vi "EX382280_Interface.vi"(7 "mode":T1, 8 "error in (no error)":errorcluster caption="에러 입력(에러 없음)", 9 "Current(A)":dbl, 10 "Voltage(V)":dbl, 11 "VISA resource name":refnum<visa-resource-name> caption="Port") -> (0 "error out":errorcluster, 3 "Read":string)   [LabVIEW 2015]
uses:
  382280_mode.ctl
  <vilib>/Instr/_visa.llb/VISA Configure Serial Port (Serial Instr).vi
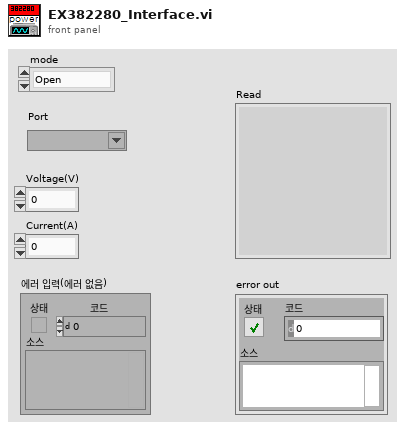
[diagram p1: front panel]
types:
  T1 = typedef "382280_mode.ctl" = enum16{"Open", "Close", "STBY", "OPER", "V SET", "A SET", "STATUS", "V Read", "A Read"}
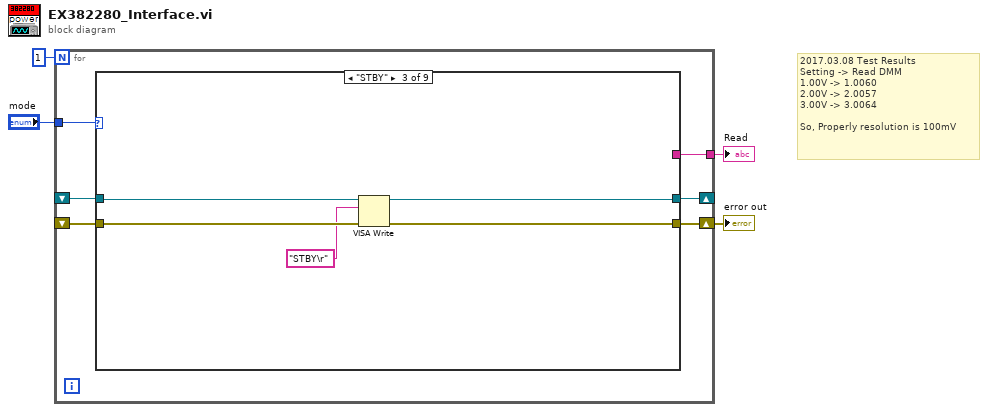
[diagram p0: block diagram]
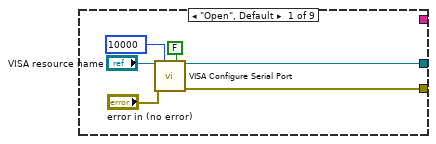
[diagram p2: hidden frame]
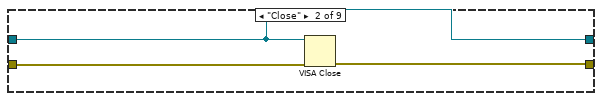
[diagram p3: hidden frame]
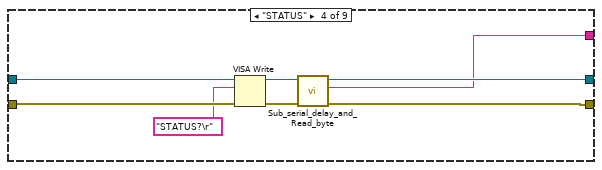
[diagram p4: hidden frame]
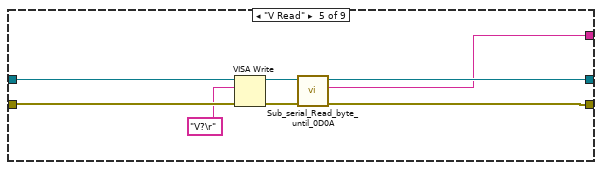
[diagram p5: hidden frame]
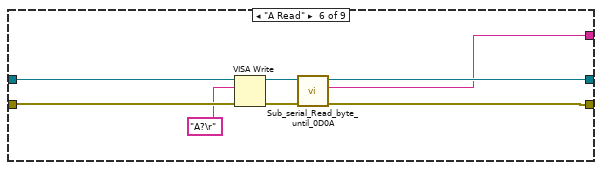
[diagram p6: hidden frame]
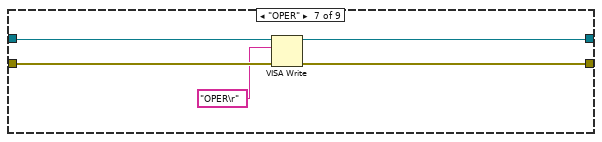
[diagram p7: hidden frame]
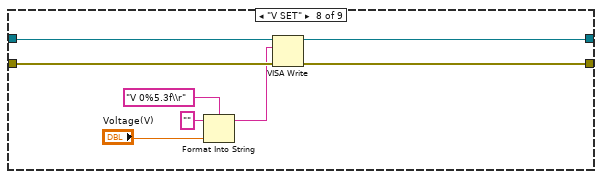
[diagram p8: hidden frame]
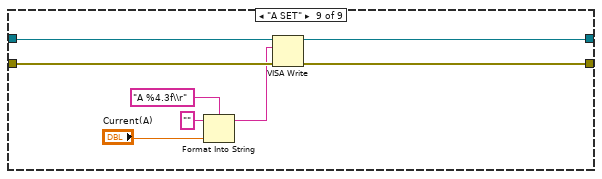
[diagram p9: hidden frame]
diagram:
  # "2017.03.08 Test Results\nSetting -> Read DMM\n1.00V -> 1.0060\n2.00V -> 2.0057 \n3.00V -> 3.0064\n\nSo, Properly resolution is 100mV"
  n1 = for {
    N: 1 -> [_]
    tunnel: "mode" -> [w10]
    shift-right: [w9] -> _
    shift-left: _ -> [w7]
    shift-right: [w8] -> w2
    shift-left: _ -> [w6]
    tunnel: [w5] -> w1
    n2 = case shown="\"STBY\"" w10 {
      tunnel: [w12 w18 w20 w32 w40 w48 w49 w56 w64] -> w9
      tunnel: [w11 w17 w22 w31 w39 w47 w51 w58 w66] -> w8
      tunnel: w7 -> [_ w18 w21 w29 w37 w45 w50 w57 w65]
      tunnel: w6 -> [_ w19 w24 w30 w38 w46 w53 w61 w69]
      tunnel: [_ _ _ w26 w34 w42 _ _ _] -> w5
      frame "Open", Default {
        n3 = call-poly "VISA Configure Serial Port"("VISA resource name"="VISA resource name", "timeout (10sec)"=u32 10000, "Enable Termination\nChar (T)"=FALSE ("Enable Termination\nChar (T)"), "error in (no error)"="error in (no error)") -> ("VISA resource name out"=w12:refnum<visa-resource-name>, "error out"=w11:errorcluster)  [unwired: 10 in]
      }
      frame "Close" {
        n4 = VISA Close(VISA resource name=w18, error in (no error)=w19) -> (error out=w17:errorcluster)
      }
      frame "STBY" {
        n5 = VISA Write(VISA resource name=w21, write buffer="STBY\r" ("버퍼 쓰기"), error in (no error)=w24) -> (VISA resource name out=w20:refnum<visa-resource-name>, error out=w22:errorcluster)  [unwired: 1 out]
      }
      frame "STATUS" {
        n6 = VISA Write(VISA resource name=w29, write buffer="STATUS?\r" ("버퍼 쓰기"), error in (no error)=w30) -> (VISA resource name out=w27:refnum<visa-resource-name>, error out=w28:errorcluster)  [unwired: 1 out]
        n7 = call "Sub_serial_delay_and_Read_byte.vi"("에러 입력(에러 없음)"=w28, "VISA 참조 번호 입력"=w27) -> ("에러 출력"=w31:errorcluster, "버퍼 읽기"=w26:string, "VISA 참조 번호 출력"=w32:refnum<visa-resource-name>)  [unwired: 7 in]
      }
      frame "V Read" {
        n8 = VISA Write(VISA resource name=w37, write buffer="V?\r" ("버퍼 쓰기"), error in (no error)=w38) -> (VISA resource name out=w35:refnum<visa-resource-name>, error out=w36:errorcluster)  [unwired: 1 out]
        n9 = call "Sub_serial_Read_byte_until_0D0A.vi"("에러 입력(에러 없음)"=w36, "VISA 참조 번호 입력"=w35) -> ("에러 출력"=w39:errorcluster, "버퍼 읽기"=w34:string, "VISA 참조 번호 출력"=w40:refnum<visa-resource-name>)  [unwired: 7 in]
      }
      frame "A Read" {
        n10 = VISA Write(VISA resource name=w45, write buffer="A?\r" ("버퍼 쓰기"), error in (no error)=w46) -> (VISA resource name out=w43:refnum<visa-resource-name>, error out=w44:errorcluster)  [unwired: 1 out]
        n11 = call "Sub_serial_Read_byte_until_0D0A.vi"("에러 입력(에러 없음)"=w44, "VISA 참조 번호 입력"=w43) -> ("에러 출력"=w47:errorcluster, "버퍼 읽기"=w42:string, "VISA 참조 번호 출력"=w48:refnum<visa-resource-name>)  [unwired: 7 in]
      }
      frame "OPER" {
        n12 = VISA Write(VISA resource name=w50, write buffer="OPER\r" ("버퍼 쓰기"), error in (no error)=w53) -> (VISA resource name out=w49:refnum<visa-resource-name>, error out=w51:errorcluster)  [unwired: 1 out]
      }
      frame "V SET" {
        n13 = Format Into String(format string="V 0%5.3f\\r" ("포맷 문자열"), initial string="" ("초기 문자열"), "Voltage(V)") -> (resulting string=w54:string)  [unwired: 1 in, 1 out]
        n14 = VISA Write(VISA resource name=w57, write buffer=w54, error in (no error)=w61) -> (VISA resource name out=w56:refnum<visa-resource-name>, error out=w58:errorcluster)  [unwired: 1 out]
      }
      frame "A SET" {
        n15 = Format Into String(format string="A %4.3f\\r" ("포맷 문자열"), initial string="" ("초기 문자열"), "Current(A)") -> (resulting string=w62:string)  [unwired: 1 in, 1 out]
        n16 = VISA Write(VISA resource name=w65, write buffer=w62, error in (no error)=w69) -> (VISA resource name out=w64:refnum<visa-resource-name>, error out=w66:errorcluster)  [unwired: 1 out]
      }
    }
  }
  "error out" <- w2
  "Read" <- w1
